vi "recursive.vi"() -> ()   [LabVIEW 2016]
panel:
  in  "Number Of Samples":i32
  in  "Amplitude":i32
  in  "Phase":i32
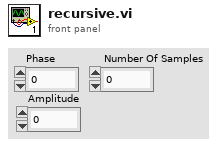
[diagram p1: front panel]
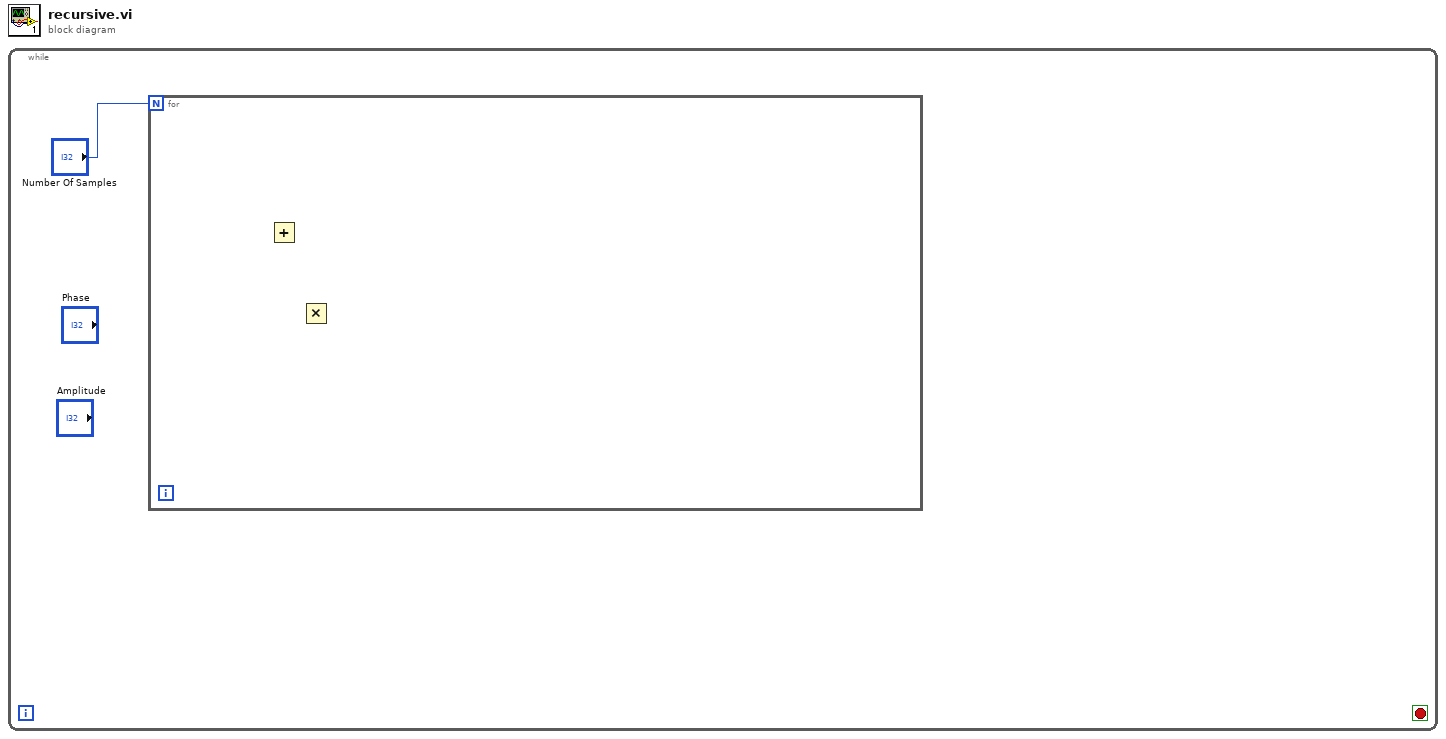
[diagram p0: block diagram]
diagram:
  n1 = while {
    stop <- _ stop-if-true
    n2 = for {
      N: "Number Of Samples" -> [_]
      n3 = Add() -> ()  [unwired: 2 in, 1 out]
      n4 = Multiply() -> ()  [unwired: 2 in, 1 out]
    }
  }
